vi "Close.vi"(8 "error in (no error)":errorcluster, 11 "Buffer Download Controller in":refnum<class "Buffer Download Controller.lvclass">) -> (0 "error out":errorcluster, 3 "Buffer Download Controller out":refnum<class "Buffer Download Controller.lvclass">)   [LabVIEW 2020, in "NI_SFTP.lvlib" / "Buffer Download Controller.lvclass"]
uses:
  <vilib>/net/SFTP/API/Support/Download/Buffer/Buffer Download Controller.lvclass
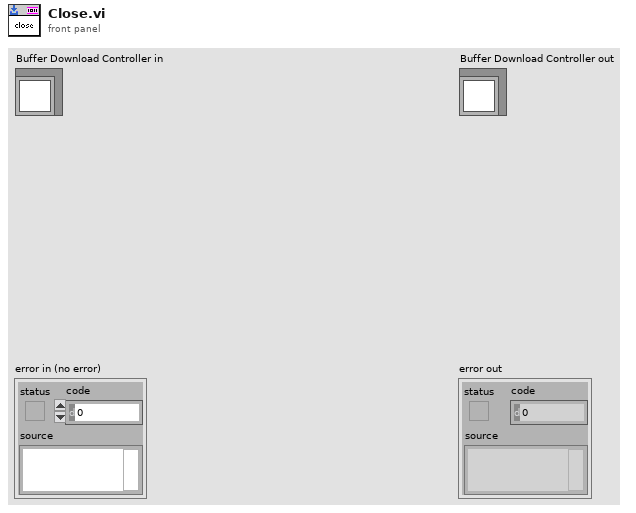
[diagram p1: front panel]
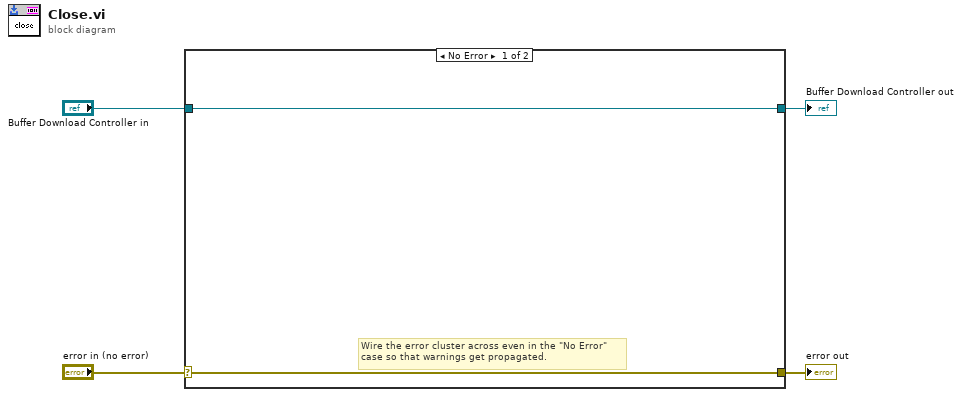
[diagram p0: block diagram]
diagram:
  n1 = case shown="No Error" "error in (no error)" {
    selector: "error in (no error)" -> [w5 w8]
    tunnel: [w5 w8] -> w3
    tunnel: [w6 w7] -> w1
    tunnel: "Buffer Download Controller in" -> [w6 w7]
    frame No Error {
      # "Wire the error cluster across even in the \"No Error\"\ncase so that warnings get propagated."
    }
    frame Error {
    }
  }
  "error out" <- w3
  "Buffer Download Controller out" <- w1
